vi "sweep.vi"(9 "Sweep Time (1.00 s)":dbl=1.0 format="%#.6g", 10 "Start Frequency (100.0 Hz)":dbl=100.0 format="%#.6g", 11 "Stop  Frequency (1000.0 Hz)":dbl=1000.0 format="%#.6g") -> ()   [LabVIEW 2016]
uses:
  <instrlib>/Agilent 33XXX Series/Agilent 33XXX Series.lvlib
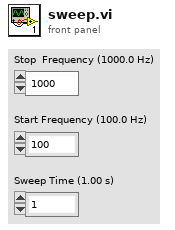
[diagram p1: front panel]
types:
  T1 = cluster{"Baud Rate":u32, "Parity":u16, "Data Bits":u16, "Flow Control":u16}
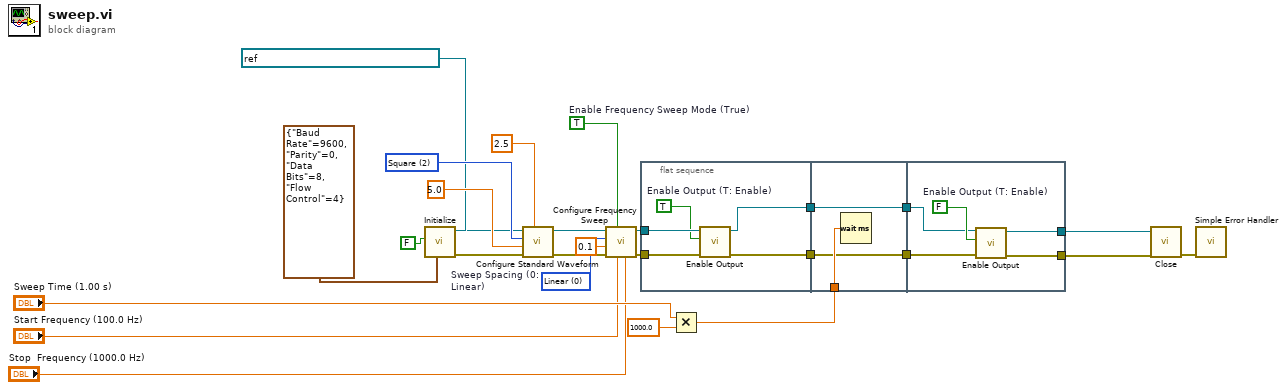
[diagram p0: block diagram]
diagram:
  w12 = u16 2 items=["DC", "Sine", "Square", "Triangle", "Ramp", "Pulse", "Noise", "Sinc", "Negative Ramp", "Exponential Rise", "Exponential Fall", "Cardiac"] ("Waveform Function (1: Sine)")
  w15 = u16 0 items=["Linear", "Logarithmic"]  # Sweep Spacing (0: Linear)
  w9 = TRUE  # Enable Frequency Sweep Mode (True)
  n1 = call <instrlib>:"Initialize.vi"("Serial Configuration"=T1 {"Baud Rate"=9600, "Parity"=0, "Data Bits"=8, "Flow Control"=4}, "ID Query (True)"=FALSE, "VISA resource name"=refnum<visa-resource-name> "TCPIP0::192.168.1.2::inst0::INSTR") -> ("error out"=w7:errorcluster, "VISA resource name out"=w2:refnum<visa-resource-name>)  [unwired: 7 in]
  n2 = call <instrlib>:"Configure Standard Waveform.vi"("DC Offset (0.00 V)"=2.5, "error in (no error)"=w7, "Amplitude (1)"=5.0 ("Amplitude (1 Vpp)"), "Waveform Function (1: Sine)"=w12, "VISA resource name"=w2) -> ("error out"=w4:errorcluster, "VISA resource name out"=w5:refnum<visa-resource-name>)  [unwired: 5 in]
  n3 = call <instrlib>:"Configure Frequency Sweep.vi"("Stop  Frequency (1000.0 Hz)"="Stop  Frequency (1000.0 Hz)", "Start Frequency (100.0 Hz)"="Start Frequency (100.0 Hz)", "Enable Frequency Sweep Mode (T: Enable)"=w9, "error in (no error)"=w4, "Sweep Time (1.00 s)"=0.1, "Sweep Spacing (0: Linear)"=w15, "VISA resource name"=w5) -> ("error out"=w14:errorcluster, "VISA resource name out"=w13:refnum<visa-resource-name>)  [unwired: 3 in]
  n4 = flat-sequence {
    tunnel: w13 -> [w32]
    tunnel: w14 -> [w31]
    tunnel: [w29] -> w27
    tunnel: [w28] -> w26
    tunnel: w21 -> [w35]
    tunnel: [w34] -> w25
    tunnel: w27 -> [w34]
    tunnel: [w33] -> w24
    tunnel: w26 -> [w33]
    tunnel: w25 -> [w39]
    tunnel: w24 -> [w38]
    tunnel: [w37] -> w22
    tunnel: [w36] -> w23
    frame #0 {
      w30 = TRUE  # Enable Output (T: Enable)
      n5 = call <instrlib>:"Enable Output.vi"("error in (no error)"=w31, "Enable Output  (T: Enable)"=w30, "VISA resource name"=w32) -> ("error out"=w28:errorcluster, "VISA resource name out"=w29:refnum<visa-resource-name>)  [unwired: 7 in]
    }
    frame #1 {
      n6 = Wait (ms)(milliseconds to wait=w35) -> ()  [unwired: 1 out]
    }
    frame #2 {
      w40 = FALSE  # Enable Output (T: Enable)
      n7 = call <instrlib>:"Enable Output.vi"("error in (no error)"=w38, "Enable Output  (T: Enable)"=w40, "VISA resource name"=w39) -> ("error out"=w36:errorcluster, "VISA resource name out"=w37:refnum<visa-resource-name>)  [unwired: 7 in]
    }
  }
  n8 = Multiply(x="Sweep Time (1.00 s)", y=1000.0) -> (x*y=w21:dbl)
  n9 = call <instrlib>:"Close.vi"("error in (no error)"=w23, "VISA resource name"=w22) -> ("error out"=w3:errorcluster)  [unwired: 9 in]
  n10 = call <vilib>:"Simple Error Handler.vi"("error in (no error)"=w3) -> ()  [unwired: 4 in, 5 out]
